vi "Read Image File (ARGB).vi"(7 "Image Read Size (Default: FULL_SIZE)":T1, 8 "error in (no error)":errorcluster, 10 "ARGB Image Destination":T2, 11 "Filepath":path) -> (0 "error out":errorcluster, 3 "ARGB Image Destination (duplicate)":T2)   [LabVIEW 2020, in "g_ar_toolkit.image.lvlib"]
uses:
  g_ar_toolkit.image.lvlib
  ARGB Image.ctl
  Image Read Size.ctl
  2358f293-6357-4b7a-bec3-c4e4d03be6e5.vi
  g_ar_toolkit.common/Module Path.vi
  <vilib>/Utility/error.llb/Error Cluster From Error Code.vi
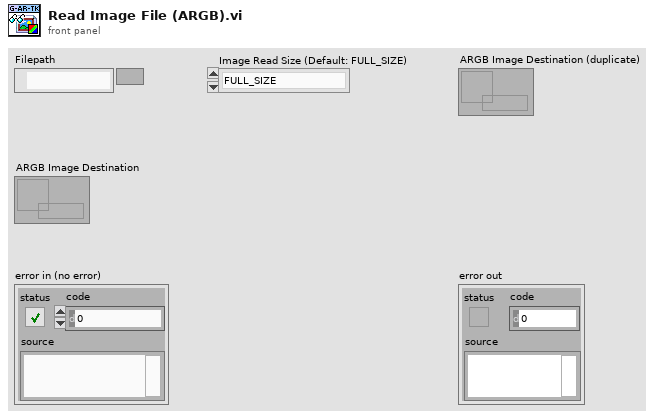
[diagram p1: front panel]
types:
  T1 = typedef "g_ar_toolkit.image.lvlib/Image Read Size.ctl" = enum8{"FULL_SIZE", "REDUCED_2", "REDUCED_4", "REDUCED_8"}
  T2 = typedef "g_ar_toolkit.image.lvlib/ARGB Image.ctl" = refnum<data-value>
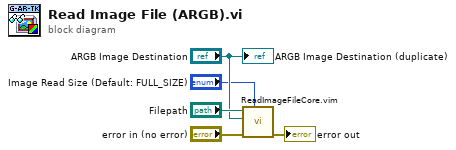
[diagram p0: block diagram]
diagram:
  n1 = call "ReadImageFileCore.vim"("Image Read Size"="Image Read Size (Default: FULL_SIZE)", "error in (no error)"="error in (no error)", "Dst"="ARGB Image Destination", "Filepath"="Filepath") -> ("error out"=→"error out":errorcluster)  [unwired: 7 in]
  "ARGB Image Destination (duplicate)" <- "ARGB Image Destination"
